vi "Read All Measurements.vi"(0 "VISA resource name":refnum<visa-resource-name>, 11 "error in (no error)":errorcluster) -> (4 "VISA resource name out":refnum<visa-resource-name>, 6 "All Measurements":T1, 15 "error out":errorcluster)   [LabVIEW 2014, in "Associated Power Technologies 8500 Series.lvlib"]
doc: "Read the all active parameter value."
uses:
  <instrlib>/Associated Power Technologies 8500 Series/Associated Power Technologies 8500 Series.lvlib
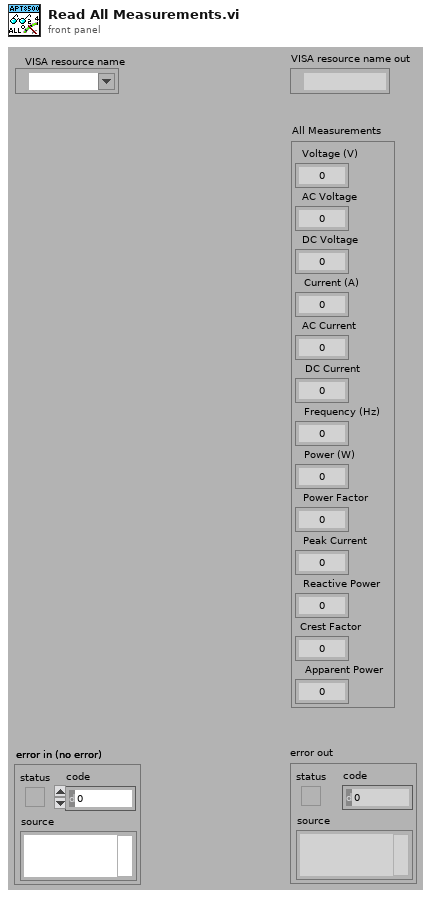
[diagram p1: front panel]
types:
  T1 = cluster{"Voltage (V)":dbl, "AC Voltage":dbl, "DC Voltage":dbl, "Current (A)":dbl, "AC Current":dbl, "DC Current":dbl, "Frequency (Hz)":dbl, "Power (W)":dbl, "Power Factor":dbl, "Peak Current":dbl, "Reactive Power":dbl, "Crest Factor":dbl, "Apparent Power":dbl}
  T2 = cluster{"Voltage (V)":dbl, "Frequency (Hz)":dbl, "Current (A)":dbl, "Power (W)":dbl, "Power Factor":dbl, "Peak Current":dbl, "Reactive Power":dbl, "Crest Factor":dbl, "Apparent Power":dbl, "AC Voltage":dbl, "AC Current":dbl, "DC Voltage":dbl, "DC Current":dbl}
  T3 = cluster{"[0]":dbl, "[1]":dbl, "[2]":dbl, "[3]":dbl, "[4]":dbl, "[5]":dbl, "[6]":dbl, "[7]":dbl, "[8]":dbl, "[9]":dbl, "[10]":dbl, "[11]":dbl, "[12]":dbl}
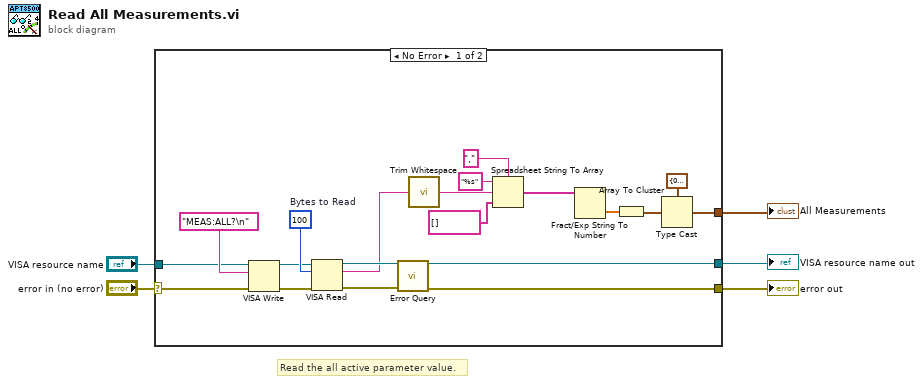
[diagram p0: block diagram]
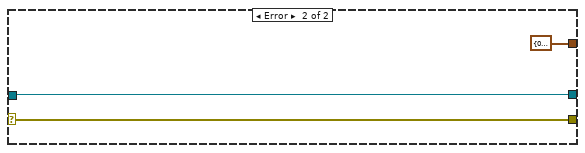
[diagram p2: hidden frame]
diagram:
  # "Read the all active parameter value."
  n1 = case shown="No Error" "error in (no error)" {
    selector: "error in (no error)" -> [w21 w28]
    tunnel: [w16 w28] -> w4
    tunnel: [w19 w27] -> w2
    tunnel: "VISA resource name" -> [w20 w27]
    tunnel: [w6 T2 {"Voltage (V)"=0.0, "Frequency (Hz)"=0.0, "Current (A)"=0.0, "Power (W)"=0.0, "Power Factor"=0.0, "Peak Current"=0.0, "Reactive Power"=0.0, "Crest Factor"=0.0, "Apparent Power"=0.0, "AC Voltage"=0.0, "AC Current"=0.0, "DC Voltage"=0.0, "DC Current"=0.0} ("All Measurements")] -> w1
    frame No Error {
      w25 = u32 100  # Bytes to Read
      n2 = VISA Write(VISA resource name=w20, write buffer="MEAS:ALL?\n", error in (no error)=w21) -> (VISA resource name out=w23:refnum<visa-resource-name>, error out=w24:errorcluster)  [unwired: 1 out]
      n3 = VISA Read(VISA resource name=w23, byte count=w25, error in (no error)=w24) -> (VISA resource name out=w18:refnum<visa-resource-name>, read buffer=w7:string, error out=w17:errorcluster)  [unwired: 1 out]
      n4 = call <instrlib>:"Error Query.vi"("VISA resource name"=w18, "error in (no error)"=w17) -> ("VISA resource name out"=w19:refnum<visa-resource-name>, "error out"=w16:errorcluster)  [unwired: 10 in, 2 out]
      n5 = call <vilib>:"Trim Whitespace.vi"("string"=w7) -> ("trimmed string"=w12:string)  [unwired: 1 in]
      n6 = Spreadsheet String To Array(delimiter (Tab)=",", format string="%s", spreadsheet string=w12, array type (2D Dbl)=string[] []) -> (array=w9:string[])
      n7 = Fract/Exp String To Number(string=w9) -> (number=w8:dbl[])  [unwired: 3 in, 1 out]
      n8 = Array To Cluster(array=w8) -> (cluster=w10:T3)
      n9 = Type Cast(type=T2 {"Voltage (V)"=0.0, "Frequency (Hz)"=0.0, "Current (A)"=0.0, "Power (W)"=0.0, "Power Factor"=0.0, "Peak Current"=0.0, "Reactive Power"=0.0, "Crest Factor"=0.0, "Apparent Power"=0.0, "AC Voltage"=0.0, "AC Current"=0.0, "DC Voltage"=0.0, "DC Current"=0.0} ("All Measurements"), x=w10) -> (*(type *) &x=w6:T2)
    }
    frame Error {
    }
  }
  "error out" <- w4
  "VISA resource name out" <- w2
  "All Measurements" <- w1
